vi "Timestamp to Timestring.vi"(11 "timestamp in":timestamp) -> (3 "time string":string)   [LabVIEW 2021, in "Game of Life.lvlib"]
doc: "This VI converts a time stamp into a time string containing date, month, year, hours, minutes and seconds in terms of microseconds."
uses:
  Game of Life.lvlib
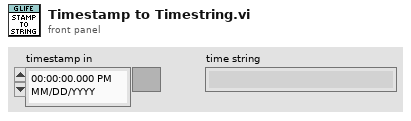
[diagram p1: front panel]
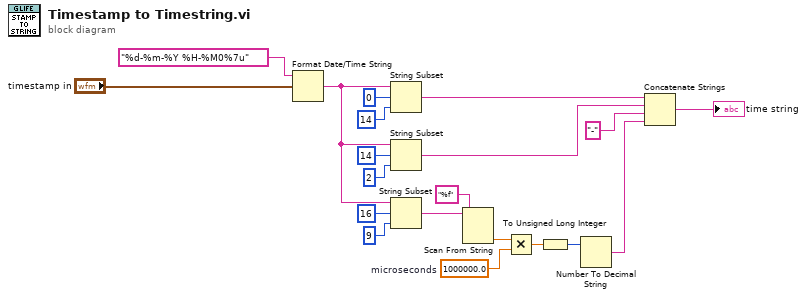
[diagram p0: block diagram]
diagram:
  w10 = 1000000.0  # microseconds
  n1 = Format Date/Time String(time format string (%c)="%d-%m-%Y %H-%M0%7u", seconds (now)="timestamp in") -> (date/time string=w7:string)  [unwired: 1 in]
  n2 = String Subset(string=w7, offset (0)=0, length (rest)=14 ("length (rest)")) -> (substring=w4:string)
  n3 = String Subset(string=w7, offset (0)=14, length (rest)=2 ("length (rest)")) -> (substring=w5:string)
  n4 = String Subset(string=w7, offset (0)=16, length (rest)=9 ("length (rest)")) -> (substring=w9:string)
  n5 = Scan From String(format string="%f", input string=w9) -> (output 1=w13:dbl)  [unwired: 3 in, 3 out]
  n6 = Multiply(x=w13, y=w10) -> (x*y=w12:dbl)
  n7 = To Unsigned Long Integer(number=w12) -> (unsigned 32bit integer=w11:u32)
  n8 = Number To Decimal String(number=w11) -> (decimal integer string=w14:string)  [unwired: 1 in]
  n9 = Concatenate Strings(w4, w5, "-" ("string"), w14) -> (→"time string":string)
